vi "Configure Cursors.vi"(0 "VISA resource name":refnum<visa-resource-name>, 1 "Target (0: Channel 1)":u16(ring) items=["Channel 1", "Channel 2", "Channel 3", "Channel 4", "Reference 1", "Reference 2", "Reference 3", "Reference 4", "Math 1", "Math 2", "Math 3", "Math 4"], 5 "Position 1 (0)":dbl, 7 "Position 2 (0)":dbl, 9 "Cursor Function (0: Cursor Off)":u16(ring) items=["Cursor Off", "Horizontal Bar Position", "Vertical Bar Position", "Paired Bar Position", "Split Bar Position", "Vertical Bar at Data Start and Stop Position"], 11 "error in (no error)":errorcluster, 12 "Time Units (0:Seconds)":u16(ring) items=["Seconds", "Hertz"], 13 "Cursor Mode (0:Independent)":u16(ring) items=["Independent", "Tracking"]) -> (4 "VISA resource name out":refnum<visa-resource-name>, 15 "error out":errorcluster)   [LabVIEW 2015, in "Tektronix 7000 Series.lvlib"]
doc: "Controls the selection of horizontal or vertical cursors, and sets cursor positions and units."
uses:
  <instrlib>/Tektronix 7000 Series/Tektronix 7000 Series.lvlib
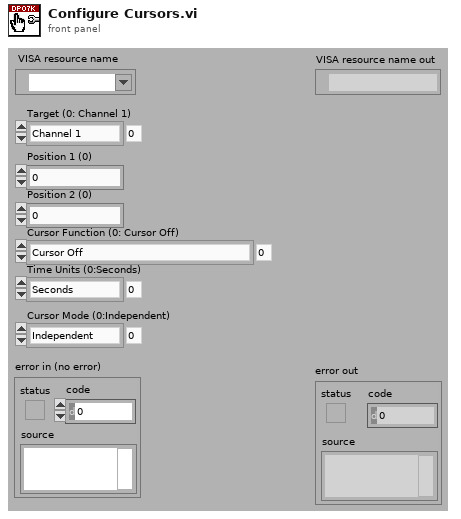
[diagram p1: front panel]
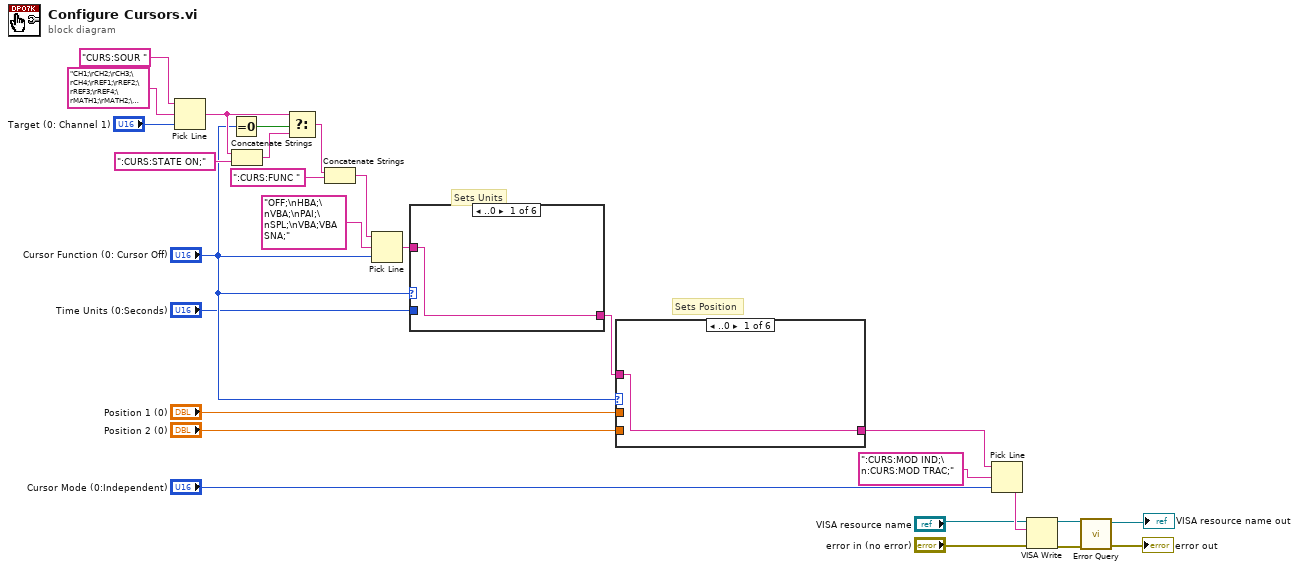
[diagram p0: block diagram]
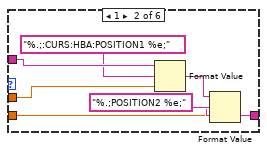
[diagram p2: hidden frame]
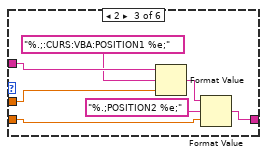
[diagram p3: hidden frame]
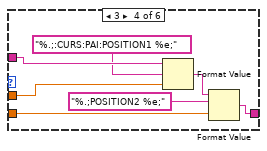
[diagram p4: hidden frame]
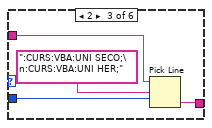
[diagram p8: hidden frame]
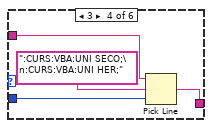
[diagram p9: hidden frame]
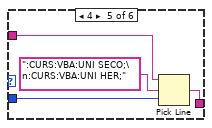
[diagram p10: hidden frame]
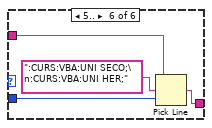
[diagram p11: hidden frame]
diagram:
  # "Sets Position"
  # "Sets Units"
  n1 = Pick Line(string ("")="CURS:SOUR ", multi-line string="CH1;\rCH2;\rCH3;\rCH4;\rREF1;\rREF2;\rREF3;\rREF4;\rMATH1;\rMATH2;\rMATH3;\nMATH4;", line index="Target (0: Channel 1)") -> (output string=w6:string)
  n2 = Equal To 0?(x="Cursor Function (0: Cursor Off)") -> (x = 0?=w8:bool)
  n3 = Concatenate Strings(w6, ":CURS:STATE ON;" ("string")) -> (w7:string)
  n4 = Select(t=w6, s=w8, f=w7) -> (s? t:f=w9:string)
  n5 = Concatenate Strings(w9, ":CURS:FUNC ") -> (w24:string)
  n6 = Pick Line(string ("")=w24, multi-line string="OFF;\nHBA;\nVBA;\nPAI;\nSPL;\nVBA;VBA SNA;", line index="Cursor Function (0: Cursor Off)") -> (output string=w10:string)
  n7 = case shown="..0" "Cursor Function (0: Cursor Off)" {
    tunnel: w10 -> [w28 w29 w33 w37 w41 w45]
    tunnel: "Time Units (0:Seconds)" -> [_ _ w31 w35 w39 w43]
    tunnel: [w28 w29 w30 w34 w38 w42] -> w11
    frame ..0 {
    }
    frame 1 {
    }
    frame 2 {
      n8 = Pick Line(string ("")=w33, multi-line string=":CURS:VBA:UNI SECO;\n:CURS:VBA:UNI HER;", line index=w31) -> (output string=w30:string)
    }
    frame 3 {
      n9 = Pick Line(string ("")=w37, multi-line string=":CURS:VBA:UNI SECO;\n:CURS:VBA:UNI HER;", line index=w35) -> (output string=w34:string)
    }
    frame 4 {
      n10 = Pick Line(string ("")=w41, multi-line string=":CURS:VBA:UNI SECO;\n:CURS:VBA:UNI HER;", line index=w39) -> (output string=w38:string)
    }
    frame 5.. {
      n11 = Pick Line(string ("")=w45, multi-line string=":CURS:VBA:UNI SECO;\n:CURS:VBA:UNI HER;", line index=w43) -> (output string=w42:string)
    }
  }
  n12 = case shown="..0" "Cursor Function (0: Cursor Off)" {
    tunnel: w11 -> [w46 w53 w60 w67 w68 w69]
    tunnel: [w46 w49 w56 w63 w68 w69] -> w20
    tunnel: "Position 1 (0)" -> [_ w48 w55 w62 _ _]
    tunnel: "Position 2 (0)" -> [_ w47 w54 w61 _ _]
    frame ..0 {
    }
    frame 1 {
      n13 = Format Value(string ("")=w53, format string="%.;:CURS:HBA:POSITION1 %e;", value (0)=w48) -> (output string=w50:string)
      n14 = Format Value(string ("")=w50, format string="%.;POSITION2 %e;", value (0)=w47) -> (output string=w49:string)
    }
    frame 2 {
      n15 = Format Value(string ("")=w60, format string="%.;:CURS:VBA:POSITION1 %e;", value (0)=w55) -> (output string=w57:string)
      n16 = Format Value(string ("")=w57, format string="%.;POSITION2 %e;", value (0)=w54) -> (output string=w56:string)
    }
    frame 3 {
      n17 = Format Value(string ("")=w67, format string="%.;:CURS:PAI:POSITION1 %e;", value (0)=w62) -> (output string=w64:string)
      n18 = Format Value(string ("")=w64, format string="%.;POSITION2 %e;", value (0)=w61) -> (output string=w63:string)
    }
    frame 4 {
    }
    frame 5.. {
    }
  }
  n19 = Pick Line(string ("")=w20, multi-line string=":CURS:MOD IND;\n:CURS:MOD TRAC;", line index="Cursor Mode (0:Independent)") -> (output string=w18:string)
  n20 = VISA Write(VISA resource name="VISA resource name", write buffer=w18, error in (no error)="error in (no error)") -> (VISA resource name out=w15:refnum<visa-resource-name>, error out=w12:errorcluster)  [unwired: 1 out]
  n21 = call <instrlib>:"Error Query.vi"("error in (no error)"=w12, "VISA resource name"=w15) -> ("error out"=→"error out":errorcluster, "VISA resource name out"=→"VISA resource name out":refnum<visa-resource-name>)  [unwired: 6 in, 2 out]
